vi "set_ref_clus_MaxiGauge.vi"(8 "input cluster":T1, 10 "value_array":dbl[](array[numeric]), 11 "error_array":errorcluster[](array[cluster])) -> ()   [LabVIEW 2019]
uses:
  cluster_ref_MaxiGauge.ctl
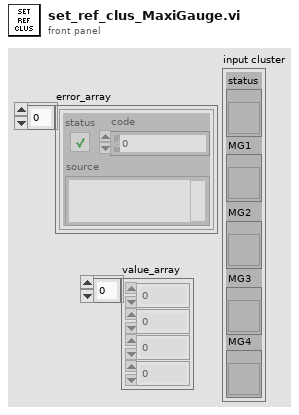
[diagram p1: front panel]
types:
  T1 = typedef "cluster_ref_MaxiGauge.ctl" = cluster{"status":refnum<vi>, "MG1":refnum<vi>, "MG2":refnum<vi>, "MG3":refnum<vi>, "MG4":refnum<vi>}
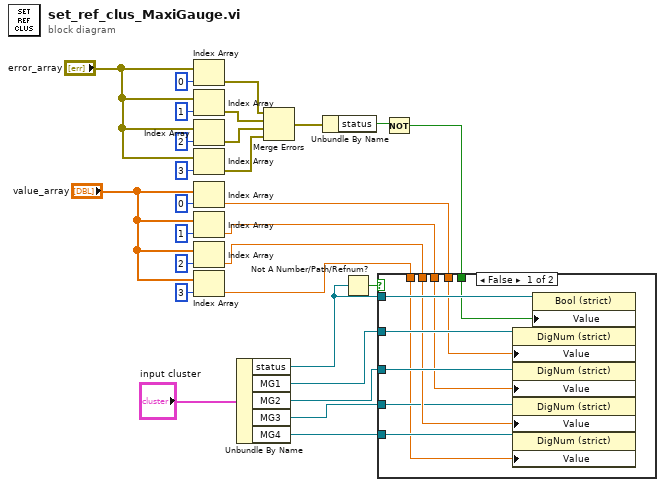
[diagram p0: block diagram]
diagram:
  n1 = Index Array(array="error_array", index=0) -> (element=w8:errorcluster)
  n2 = Index Array(array="error_array", index=1) -> (element=w6:errorcluster)
  n3 = Index Array(array="error_array", index=2) -> (element=w5:errorcluster)
  n4 = Index Array(array="error_array", index=3) -> (element=w4:errorcluster)
  n5 = Index Array(array="value_array", index=0) -> (element=w20:dbl)
  n6 = Index Array(array="value_array", index=1) -> (element=w15:dbl)
  n7 = Index Array(array="value_array", index=2) -> (element=w14:dbl)
  n8 = Index Array(array="value_array", index=3) -> (element=w13:dbl)
  n9 = Unbundle By Name("input cluster") -> ("status"=w25:refnum<vi>, "MG1"=w26:refnum<vi>, "MG2"=w27:refnum<vi>, "MG3"=w24:refnum<vi>, "MG4"=w22:refnum<vi>)
  n10 = Merge Errors(w8, w6, w5, w4) -> (w3:errorcluster)
  n11 = Unbundle By Name(w3) -> ("status"=w2:bool)
  n12 = Not A Number/Path/Refnum?(number/path/refnum=w25) -> (NaN/Path/Refnum?=w28:bool)
  n13 = Not(x=w2) -> (.not. x?=w1:bool)
  n14 = case shown="False" w28 {
    tunnel: w26 -> [w38 _]
    tunnel: w27 -> [w37 _]
    tunnel: w25 -> [w36 _]
    tunnel: w1 -> [w35 _]
    tunnel: w20 -> [w34 _]
    tunnel: w15 -> [w33 _]
    tunnel: w14 -> [w32 _]
    tunnel: w24 -> [w31 _]
    tunnel: w22 -> [w30 _]
    tunnel: w13 -> [w29 _]
    frame False {
      n15 = property class="DigNum (strict)"(reference=w38, "Value"=w34) -> ()  [unwired: 1 in, 2 out]
      n16 = property class="DigNum (strict)"(reference=w37, "Value"=w33) -> ()  [unwired: 1 in, 2 out]
      n17 = property class="DigNum (strict)"(reference=w31, "Value"=w32) -> ()  [unwired: 1 in, 2 out]
      n18 = property class="DigNum (strict)"(reference=w30, "Value"=w29) -> ()  [unwired: 1 in, 2 out]
      n19 = property class="Bool (strict)"(reference=w36, "Value"=w35) -> ()  [unwired: 1 in, 2 out]
    }
    frame True {
    }
  }
